vi "Peak detector.vi"(5 "X":cdb[](array[numeric]), 9 "Y":cdb[](array[numeric])) -> (6 "peak\nvalue":dbl, 8 "peak\nindex":i32, 10 "r":dbl[](array[numeric]))   [LabVIEW 2017]
uses:
  <vilib>/Analysis/2dsp.llb/Complex FFT.vi
  <vilib>/Analysis/2dsp.llb/Inverse Complex FFT.vi
  <vilib>/Analysis/NI_AALPro.lvlib
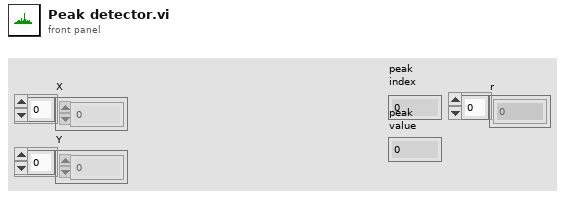
[diagram p1: front panel]
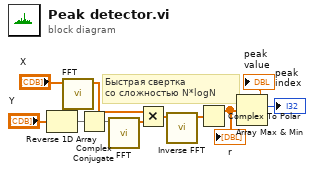
[diagram p0: block diagram]
diagram:
  # "Быстрая свертка \nсо сложностью N*logN"
  n1 = Reverse 1D Array(array="Y") -> (reversed array=w5:cdb[])
  n2 = call-poly <vilib>:"FFT.vi"("X"="X") -> ("FFT {X}"=w9:cdb[])  [unwired: 9 in, 1 out]
  n3 = Complex Conjugate(1:w5) -> (0:w10:cdb[])
  n4 = call-poly <vilib>:"FFT.vi"("X"=w10) -> ("FFT {X}"=w8:cdb[])  [unwired: 9 in, 1 out]
  n5 = Multiply(x=w9, y=w8) -> (x*y=w7:cdb[])
  n6 = call-poly <vilib>:"Inverse FFT.vi"("FFT {X}"=w7) -> ("X"=w4:cdb[])  [unwired: 9 in, 1 out]
  n7 = Complex To Polar(r * e^(i*theta)=w4) -> (r=w1:dbl[])  [unwired: 1 out]
  "r" <- w1
  n8 = Array Max & Min(array=w1) -> (max value=→"peak\nvalue":dbl, max index (indices)=→"peak\nindex":i32)  [unwired: 2 out]
